vi "Configure PID Scheduler Boundary Parameters.vi"(7 "Unit Address (1)":u8=1, 8 "error in (no error)":errorcluster, 9 "Scheduler Boundary 2-3 (0)":i32, 10 "Scheduler Boundary 1-2 (0)":i32, 11 "VISA resource name":refnum<visa-resource-name>) -> (0 "error out":errorcluster, 3 "VISA resource name out":refnum<visa-resource-name>)   [LabVIEW 2014, in "Eurotherm 35xx Series.lvlib"]
doc: "This VI sets PID Scheduler Boundary parameters."
uses:
  <instrlib>/Eurotherm 35xx Series/Eurotherm 35xx Series.lvlib
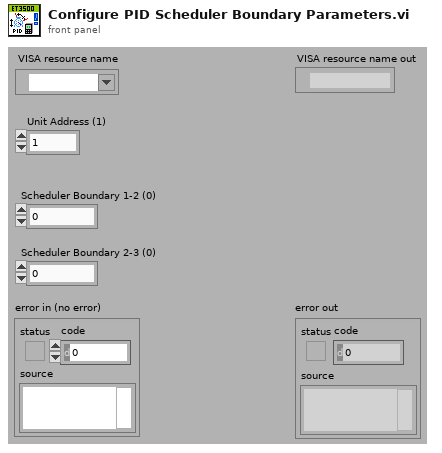
[diagram p1: front panel]
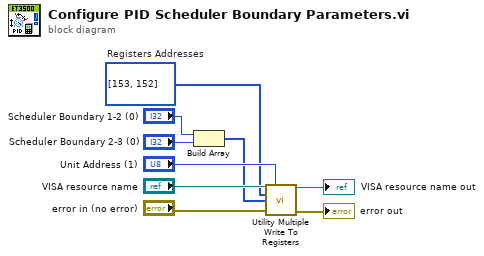
[diagram p0: block diagram]
diagram:
  w1 = u16[] [153, 152]  # Registers Addresses
  n1 = Build Array("Scheduler Boundary 1-2 (0)", "Scheduler Boundary 2-3 (0)") -> (w2:i32[])
  n2 = call <instrlib>:"Utility Multiple Write To Registers.vi"("VISA resource name"="VISA resource name", "Unit Address (1)"="Unit Address (1)", "Registers Addresses (0)"=w1, "Data (0)"=w2, "error in (no error)"="error in (no error)") -> ("VISA resource name out"=→"VISA resource name out":refnum<visa-resource-name>, "error out"=→"error out":errorcluster)  [unwired: 9 in]
